vi "TXRefNew.vi"(8 "error in (no error)":errorcluster caption="错误输入（无错误）", 10 "通讯接口数据":T1, 11 "MainPage 输入":refnum<class "MainPage.lvclass">) -> (0 "error out":errorcluster caption="错误输出", 2 "通讯接口引用":refnum<data-value>, 3 "MainPage 输出":refnum<class "MainPage.lvclass">)   [LabVIEW 2019, in "MainPage.lvlib" / "MainPage.lvclass"]
uses:
  MainPage.lvclass
  MainPage.lvclass/MainPage.ctl
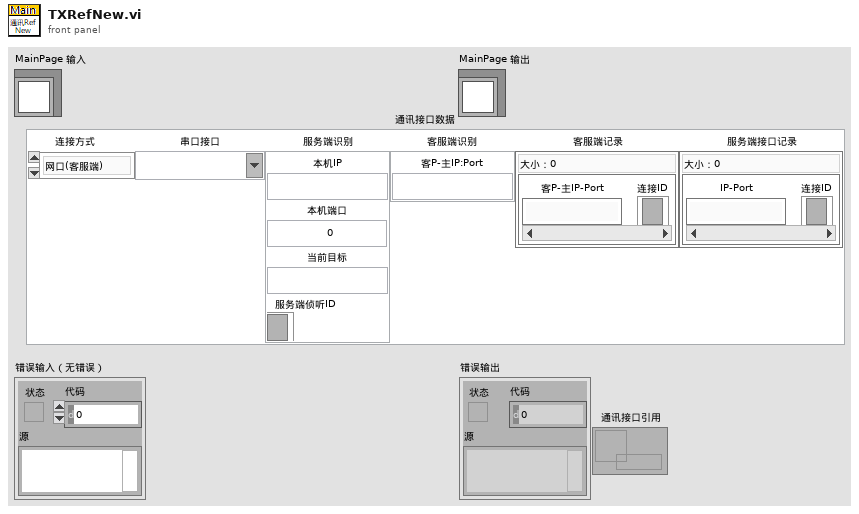
[diagram p1: front panel]
types:
  T1 = typedef "MainPage.lvlib/MainPage.lvclass/DataRef_通讯接口.ctl" = cluster{"连接方式":enum16{"网口(客服端)", "网口(服务端)", "串口"}, "VISA串口名称":refnum<visa-resource-name>, "服务端识别":cluster{"本机IP":string, "本机端口":u16, "当前目标":string, "服务端侦听ID":refnum<k5>}, "客服端识别":cluster{"客P-主IP:Port":string}, "客服端记录":map{string, refnum<k5>}, "服务端接口记录":map{string, refnum<k5>}}
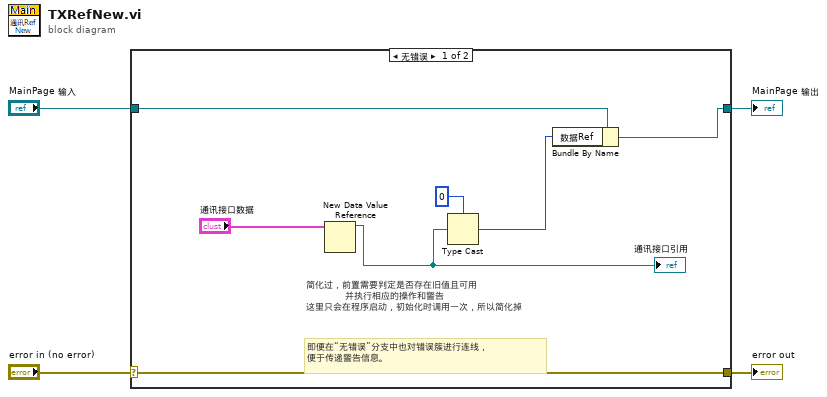
[diagram p0: block diagram]
diagram:
  n1 = case shown="无错误" "error in (no error)" {
    selector: "error in (no error)" -> [w11 w13]
    tunnel: [w11 w13] -> w3
    tunnel: [w8 w12] -> w1
    tunnel: "MainPage 输入" -> [w9 w12]
    frame No Error {
      # "简化过，前置需要判定是否存在旧值且可用\n             并执行相应的操作和警告\n这里只会在程序启动，初始化时调用一次，所以简化掉"
      # "即便在“无错误”分支中也对错误簇进行连线，\n便于传递警告信息。"
      n2 = New Data Value Reference(data value="通讯接口数据") -> (data value reference=w7:refnum<data-value>)  [unwired: 1 in, 1 out]
      "通讯接口引用" <- w7
      n3 = Type Cast(type=u32 0 ("DataRef"), x=w7) -> (*(type *) &x=w5:u32)
      n4 = Bundle By Name(cluster=w9, "数据Ref"=w5) -> (w8:refnum<class "MainPage.lvclass">)
    }
    frame Error {
    }
  }
  "error out" <- w3
  "MainPage 输出" <- w1
